vi "Autonomous Independent.vi"   [LabVIEW 2023]
doc: "This VI is called when autonomous begins, and will automatically be terminated when autonomous ends. You can carry out timed or sensor driven robot movement independently without needing to return to the caller."
uses:
  Shoulder/ShoulderGetSetpointEnum.ctl
  Auton Main/State Machine/Auot FIFO.ctl
  Auton Main/Auton Main Array.ctl
  Auton Main/State Machine/FIFO Array.ctl
  <vilib>/Rock Robotics/WPI/ThirdParty/JAS_Junk/TrajLib/Trajectory_Library.lvlib
  Auton Main/State Machine/Auot States.ctl
  Trajectory/TrajectoryGlobals.vi
  <vilib>/Rock Robotics/Network Tables/NT Read String.vi
  <vilib>/Rock Robotics/Network Tables/NT Write Number.vi
panel:
  # "Be sure to right-click and choose Data Operations>>Make Current Value default if you want to save the array values with the VI"
types:
  T1 = typedef "ShoulderGetSetpointEnum.ctl" = enum16{"Select", "ShoulderRest", "ShoulderSpeaker", "ShoulderAmp"}
  T2 = typedef "Auot States.ctl" = enum16{"Unknown", "Initilize", "Intake", "Move Arm", "Drive Straight", "Drive Trajorctory", "Drive Turn", "Send Bool CMD", "Set Target", "Shoot", "Wait", "Exit"}
  T3 = typedef "FIFO Array.ctl" = T4[]
  T4 = typedef "Auot FIFO.ctl" = cluster{"Auto States":T2, "Dist":dbl, "Radians":dbl, "MaxSpeed (ft/s)":dbl, "TimeOut (s)":dbl, "CMD":string, "ArmSetpoints":T1}
  T5 = typedef "Auton Main Array.ctl" = cluster{"FIFO Array":T3, "Dist (ft)":dbl, "MaxSpeed (ft/s)":dbl, "TimeOut (s)":dbl, "Timer Value":u32, "DriveStraightDistance":dbl[], "ModuleTravelPosition":dbl[], "First Time":bool, "Current Step":T4}
  T6 = typedef "Trajectory_Library.lvlib/TRAJECTORY.ctl" = cluster{"TotalTImeSecs":dbl, "States":T7[]}
  T7 = typedef "Trajectory_Library.lvlib/TRAJ_STATE.ctl" = cluster{"TimeSeconds":dbl, "Velocity":dbl, "Acceleration":dbl, "POSE":T8, "Curvature":dbl}
  T8 = typedef "Trajectory_Library.lvlib/POSE2D.ctl" = cluster{"TRANSLATION":T9, "ROTATION":T10}
  T9 = typedef "Trajectory_Library.lvlib/TRANSLATION2D.ctl" = cluster{"X":dbl, "Y":dbl}
  T10 = typedef "Trajectory_Library.lvlib/ROTATION2D.ctl" = cluster{"VALUE":dbl, "COS":dbl, "SIN":dbl}
  T11 = typedef "Trajectory_Library.lvlib/CHASSIS_SPEEDS.ctl" = cluster{"vX":dbl, "vY":dbl, "vOmega":dbl}
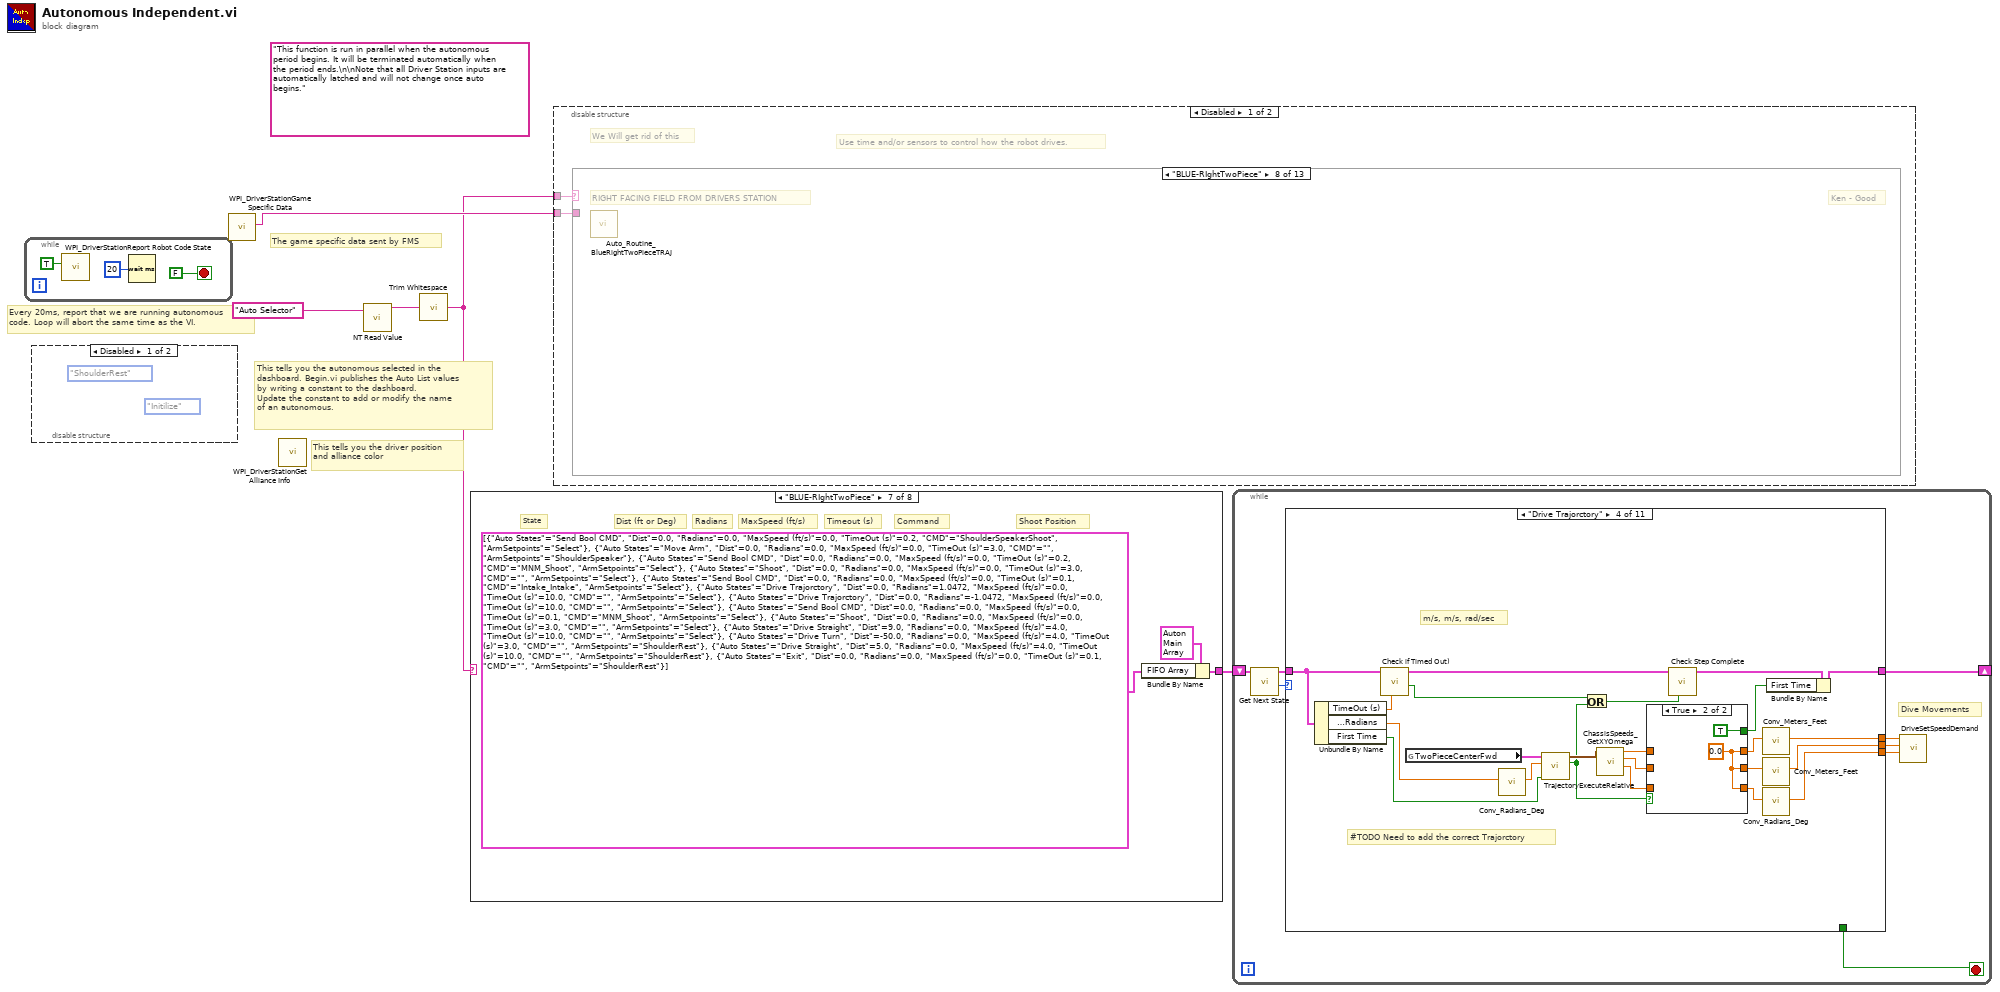
[diagram p0: block diagram]
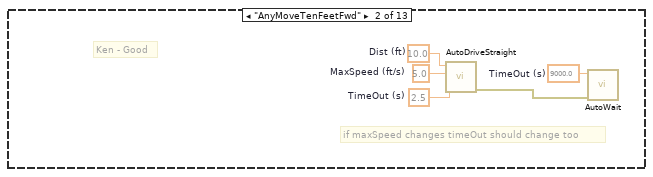
[diagram p3: hidden frame]
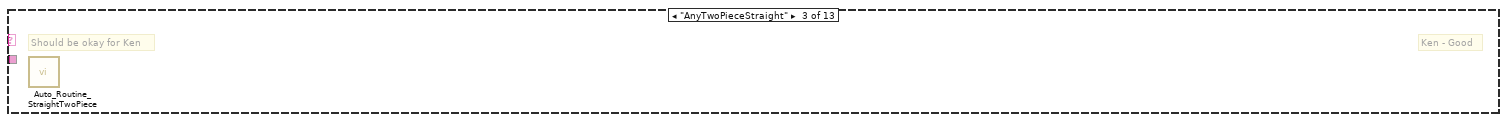
[diagram p4: hidden frame]
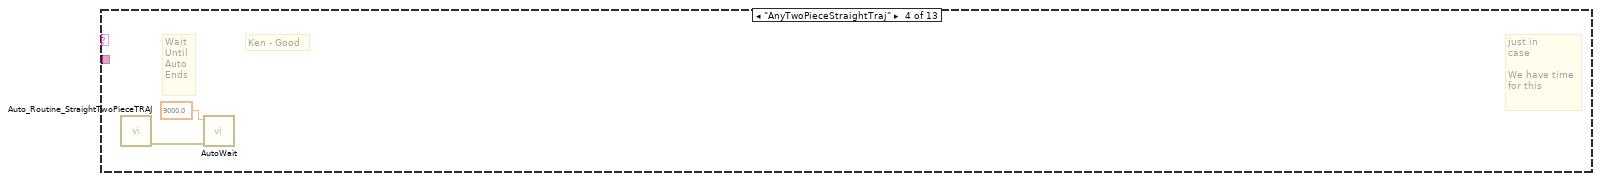
[diagram p5: hidden frame]
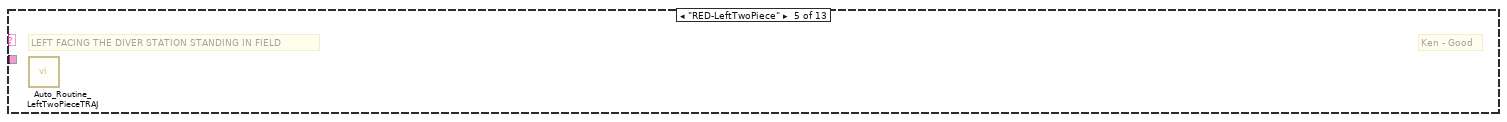
[diagram p6: hidden frame]
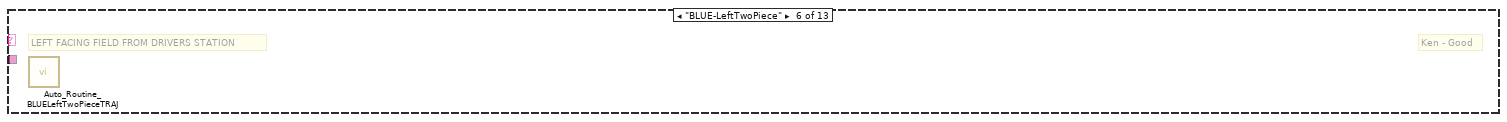
[diagram p7: hidden frame]
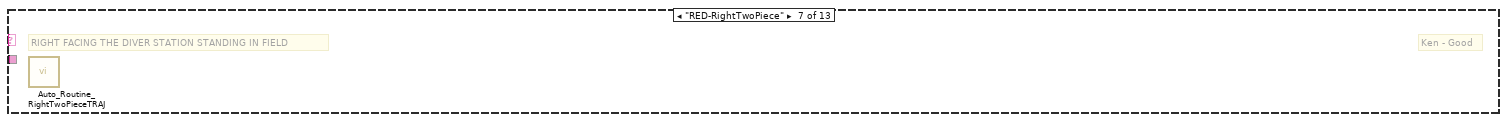
[diagram p8: hidden frame]
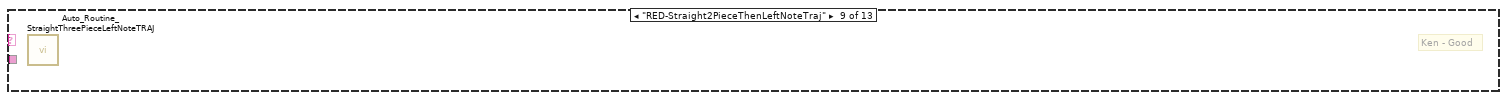
[diagram p9: hidden frame]
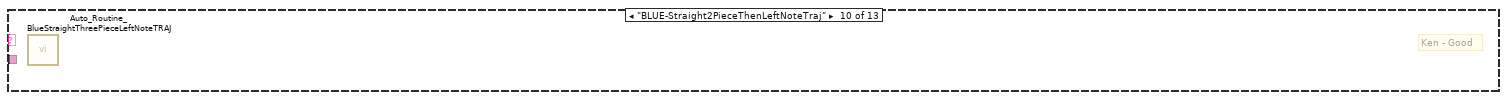
[diagram p10: hidden frame]
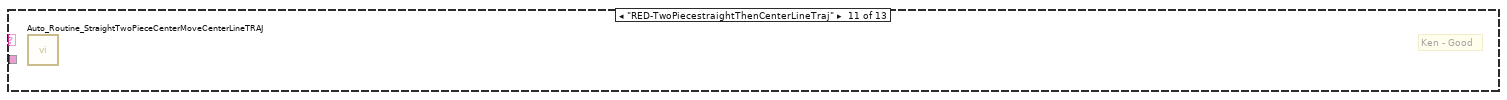
[diagram p11: hidden frame]
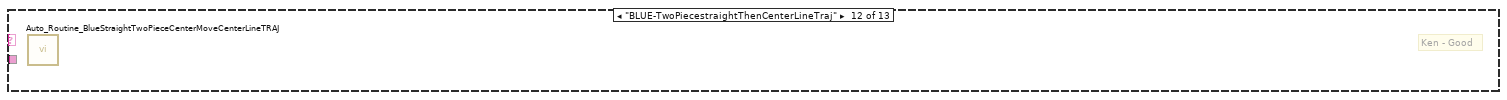
[diagram p12: hidden frame]
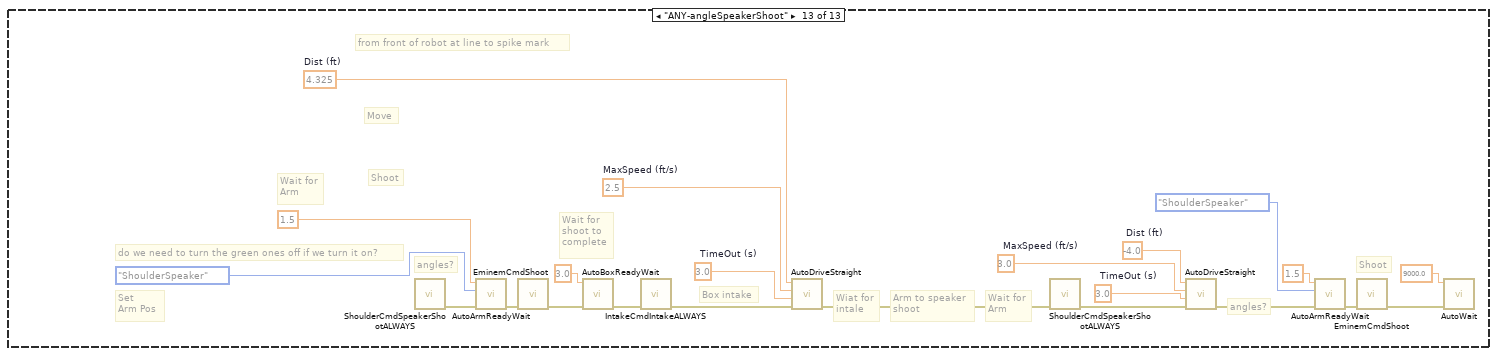
[diagram p13: hidden frame]
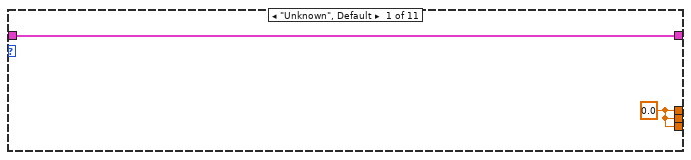
[diagram p16: hidden frame]
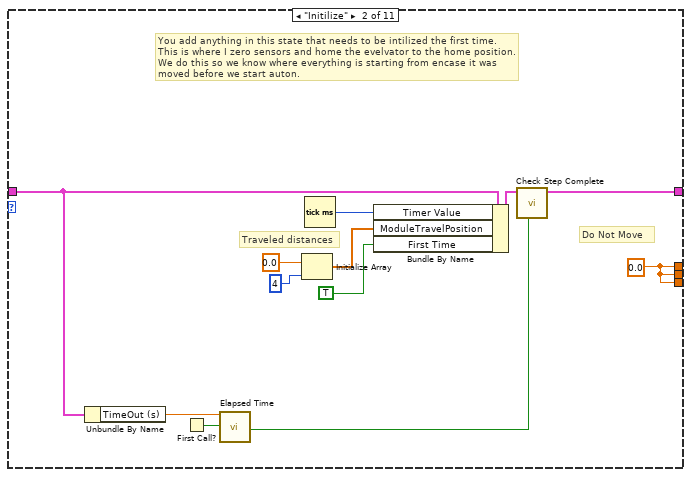
[diagram p17: hidden frame]
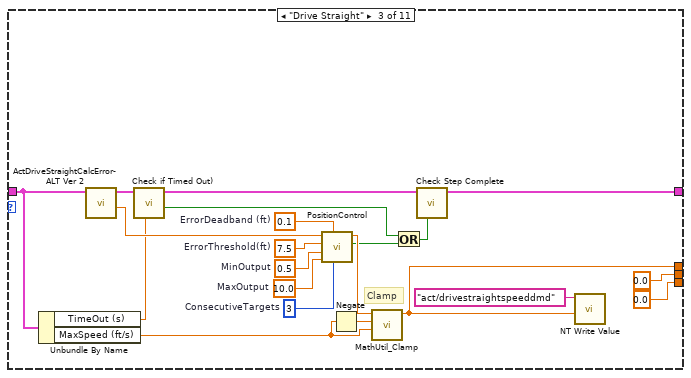
[diagram p18: hidden frame]
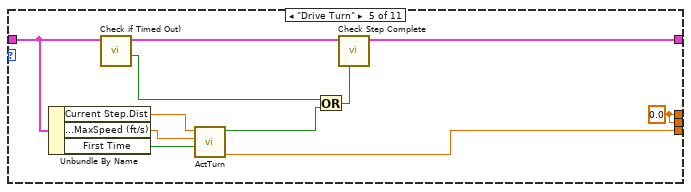
[diagram p20: hidden frame]
diagram:
  (unwired) "This function is run in parallel when the autonomous period begins. It will be terminated automatically when the period ends.\n\nNote that all Driver Station inputs are automatically latched and will not change once auto begins."
  # "The game specific data sent by FMS"
  # "This tells you the autonomous selected in the \ndashboard. Begin.vi publishes the Auto List values\nby writing a constant to the dashboard.\nUpdate the constant to add or modify the name\nof an autonomous."
  # "Every 20ms, report that we are running autonomous\ncode. Loop will abort the same time as the VI."
  # "This tells you the driver position\nand alliance color"
  n1 = while {
    stop <- FALSE stop-if-true
    n2 = call <vilib>:"WPI_DriverStationReport Robot Code State.vi"("Autonomous"=TRUE) -> ()  [unwired: 10 in, 1 out]
    n3 = Wait (ms)(milliseconds to wait=u32 20) -> ()  [unwired: 1 out]
  }
  n4 = disable-structure shown="Disabled" {
    frame Disabled {
      (unwired) ShoulderGetSetpointEnum."ShoulderRest" ("ArmSetpoints")
      (unwired) Auot_States."Initilize" ("Auto States")
    }
    frame Enabled {
    }
  }
  n5 = call <vilib>:"WPI_DriverStationGame Specific Data.vi"() -> ("Game Specific Data"=w4:string)  [unwired: 11 in]
  n6 = call <vilib>:"WPI_DriverStationGet Alliance Info.vi"() -> ()  [unwired: 12 out]
  n7 = call-poly <vilib>:"NT Read Value.vi"("name"="Auto Selector" ("Name")) -> ("value"=w3:string)  [unwired: 8 in, 2 out]
  n8 = call <vilib>:"Trim Whitespace.vi"("string"=w3) -> ("trimmed string"=w2:string)  [unwired: 1 in]
  n9 = case shown="\"BLUE-RIghtTwoPiece\"" w2 {
    tunnel: [w10 w13 w16 w19 w22 w25 w28 T5 {"FIFO Array"=[{"Auto States"=enum."Initilize", "Dist"=4.3, "Radians"=0.0, "MaxSpeed (ft/s)"=1.2, "TimeOut (s)"=10.0, "CMD"="", "ArmSetpoints"=enum."Select"}], "Dist (ft)"=0.0, "MaxSpeed (ft/s)"=0.0, "TimeOut (s)"=99.0, "Timer Value"=0, "DriveStraightDistance"=[], "ModuleTravelPosition"=[], "First Time"=FALSE, "Current Step"={"Auto States"=enum."Unknown", "Dist"=4.3, "Radians"=0.0, "MaxSpeed (ft/s)"=1.2, "TimeOut (s)"=10.0, "CMD"="", "ArmSetpoints"=enum."ShoulderRest"}} ("Main Array")] -> w1
    frame "AnyMoveTenFeetFwd" {
      # "Radians"
      # "Shoot Position"
      # "Command"
      # "Timeout (s)"
      # "MaxSpeed (ft/s)"
      # "Dist (ft)"
      # "State"
      n10 = Bundle By Name(cluster=T5 {"FIFO Array"=[{"Auto States"=enum."Initilize", "Dist"=4.3, "Radians"=0.0, "MaxSpeed (ft/s)"=1.2, "TimeOut (s)"=10.0, "CMD"="", "ArmSetpoints"=enum."ShoulderRest"}], "Dist (ft)"=0.0, "MaxSpeed (ft/s)"=0.0, "TimeOut (s)"=99.0, "Timer Value"=0, "DriveStraightDistance"=[], "ModuleTravelPosition"=[0.0, 0.0, 0.0, 0.0], "First Time"=FALSE, "Current Step"={"Auto States"=enum."Unknown", "Dist"=4.3, "Radians"=0.0, "MaxSpeed (ft/s)"=1.2, "TimeOut (s)"=10.0, "CMD"="", "ArmSetpoints"=enum."ShoulderRest"}} ("Main Array"), "FIFO Array"=T3 [{"Auto States"=enum."Initilize", "Dist"=0.0, "Radians"=0.0, "MaxSpeed (ft/s)"=0.0, "TimeOut (s)"=1.0, "CMD"="", "ArmSetpoints"=enum."Select"}, {"Auto States"=enum."Drive Straight", "Dist"=10.0, "Radians"=0.0, "MaxSpeed (ft/s)"=5.0, "TimeOut (s)"=2.5, "CMD"="", "ArmSetpoints"=enum."Select"}, {"Auto States"=enum."Exit", "Dist"=0.0, "Radians"=0.0, "MaxSpeed (ft/s)"=0.0, "TimeOut (s)"=0.1, "CMD"="", "ArmSetpoints"=enum."Select"}]) -> (w10:T5)
    }
    frame "AnyTwoPieceStraight" {
      # "Radians"
      # "Shoot Position"
      # "Command"
      # "Timeout (s)"
      # "MaxSpeed (ft/s)"
      # "Dist (ft)"
      # "State"
      n11 = Bundle By Name(cluster=T5 {"FIFO Array"=[{"Auto States"=enum."Initilize", "Dist"=0.0, "Radians"=0.0, "MaxSpeed (ft/s)"=0.0, "TimeOut (s)"=0.0, "CMD"="", "ArmSetpoints"=enum."ShoulderRest"}], "Dist (ft)"=0.0, "MaxSpeed (ft/s)"=0.0, "TimeOut (s)"=99.0, "Timer Value"=0, "DriveStraightDistance"=[], "ModuleTravelPosition"=[0.0, 0.0, 0.0, 0.0], "First Time"=FALSE, "Current Step"={"Auto States"=enum."Unknown", "Dist"=4.3, "Radians"=0.0, "MaxSpeed (ft/s)"=1.2, "TimeOut (s)"=10.0, "CMD"="", "ArmSetpoints"=enum."ShoulderRest"}} ("Main Array"), "FIFO Array"=T3 [{"Auto States"=enum."Initilize", "Dist"=0.0, "Radians"=0.0, "MaxSpeed (ft/s)"=0.0, "TimeOut (s)"=1.0, "CMD"="", "ArmSetpoints"=enum."Select"}, {"Auto States"=enum."Send Bool CMD", "Dist"=0.0, "Radians"=0.0, "MaxSpeed (ft/s)"=0.0, "TimeOut (s)"=0.2, "CMD"="ShoulderSpeakerShoot", "ArmSetpoints"=enum."Select"}, {"Auto States"=enum."Move Arm", "Dist"=0.0, "Radians"=0.0, "MaxSpeed (ft/s)"=0.0, "TimeOut (s)"=0.5, "CMD"="", "ArmSetpoints"=enum."ShoulderSpeaker"}, {"Auto States"=enum."Send Bool CMD", "Dist"=0.0, "Radians"=0.0, "MaxSpeed (ft/s)"=0.0, "TimeOut (s)"=0.2, "CMD"="MNM_Shoot", "ArmSetpoints"=enum."Select"}, {"Auto States"=enum."Shoot", "Dist"=0.0, "Radians"=0.0, "MaxSpeed (ft/s)"=0.0, "TimeOut (s)"=3.0, "CMD"="", "ArmSetpoints"=enum."Select"}, {"Auto States"=enum."Send Bool CMD", "Dist"=0.0, "Radians"=0.0, "MaxSpeed (ft/s)"=0.0, "TimeOut (s)"=0.2, "CMD"="Intake_Intake", "ArmSetpoints"=enum."Select"}, {"Auto States"=enum."Drive Straight", "Dist"=4.3, "Radians"=0.0, "MaxSpeed (ft/s)"=1.2, "TimeOut (s)"=10.0, "CMD"="", "ArmSetpoints"=enum."Select"}, {"Auto States"=enum."Drive Straight", "Dist"=-4.0, "Radians"=0.0, "MaxSpeed (ft/s)"=3.0, "TimeOut (s)"=3.0, "CMD"="", "ArmSetpoints"=enum."Select"}, {"Auto States"=enum."Send Bool CMD", "Dist"=0.0, "Radians"=0.0, "MaxSpeed (ft/s)"=0.0, "TimeOut (s)"=0.2, "CMD"="MNM_Shoot", "ArmSetpoints"=enum."Select"}, {"Auto States"=enum."Shoot", "Dist"=0.0, "Radians"=0.0, "MaxSpeed (ft/s)"=0.0, "TimeOut (s)"=3.0, "CMD"="", "ArmSetpoints"=enum."Select"}, {"Auto States"=enum."Drive Straight", "Dist"=4.0, "Radians"=0.0, "MaxSpeed (ft/s)"=3.0, "TimeOut (s)"=8.0, "CMD"="", "ArmSetpoints"=enum."Select"}, {"Auto States"=enum."Exit", "Dist"=0.0, "Radians"=0.0, "MaxSpeed (ft/s)"=0.0, "TimeOut (s)"=0.1, "CMD"="", "ArmSetpoints"=enum."Select"}]) -> (w13:T5)
    }
    frame "AnyTwoPieceStraightTraj" {
      # "Radians"
      # "Shoot Position"
      # "Command"
      # "Timeout (s)"
      # "MaxSpeed (ft/s)"
      # "Dist (ft)"
      # "State"
      n12 = Bundle By Name(cluster=T5 {"FIFO Array"=[{"Auto States"=enum."Initilize", "Dist"=0.0, "Radians"=0.0, "MaxSpeed (ft/s)"=0.0, "TimeOut (s)"=0.0, "CMD"="", "ArmSetpoints"=enum."ShoulderRest"}], "Dist (ft)"=0.0, "MaxSpeed (ft/s)"=0.0, "TimeOut (s)"=99.0, "Timer Value"=0, "DriveStraightDistance"=[], "ModuleTravelPosition"=[0.0, 0.0, 0.0, 0.0], "First Time"=FALSE, "Current Step"={"Auto States"=enum."Unknown", "Dist"=4.3, "Radians"=0.0, "MaxSpeed (ft/s)"=1.2, "TimeOut (s)"=10.0, "CMD"="", "ArmSetpoints"=enum."ShoulderRest"}} ("Main Array"), "FIFO Array"=T3 [{"Auto States"=enum."Initilize", "Dist"=0.0, "Radians"=0.0, "MaxSpeed (ft/s)"=0.0, "TimeOut (s)"=0.1, "CMD"="", "ArmSetpoints"=enum."Select"}, {"Auto States"=enum."Send Bool CMD", "Dist"=0.0, "Radians"=0.0, "MaxSpeed (ft/s)"=0.0, "TimeOut (s)"=0.2, "CMD"="ShoulderSpeakerShoot", "ArmSetpoints"=enum."Select"}, {"Auto States"=enum."Send Bool CMD", "Dist"=0.0, "Radians"=0.0, "MaxSpeed (ft/s)"=0.0, "TimeOut (s)"=0.2, "CMD"="MNM_ShootRev", "ArmSetpoints"=enum."Select"}, {"Auto States"=enum."Move Arm", "Dist"=0.0, "Radians"=0.0, "MaxSpeed (ft/s)"=0.0, "TimeOut (s)"=1.5, "CMD"="", "ArmSetpoints"=enum."ShoulderSpeaker"}, {"Auto States"=enum."Send Bool CMD", "Dist"=0.0, "Radians"=0.0, "MaxSpeed (ft/s)"=0.0, "TimeOut (s)"=0.2, "CMD"="MNM_Shoot", "ArmSetpoints"=enum."Select"}, {"Auto States"=enum."Shoot", "Dist"=0.0, "Radians"=0.0, "MaxSpeed (ft/s)"=0.0, "TimeOut (s)"=3.0, "CMD"="", "ArmSetpoints"=enum."Select"}, {"Auto States"=enum."Send Bool CMD", "Dist"=0.0, "Radians"=0.0, "MaxSpeed (ft/s)"=0.0, "TimeOut (s)"=0.2, "CMD"="Intake_Intake", "ArmSetpoints"=enum."Select"}, {"Auto States"=enum."Drive Trajorctory", "Dist"=0.0, "Radians"=0.0, "MaxSpeed (ft/s)"=0.0, "TimeOut (s)"=10.0, "CMD"="", "ArmSetpoints"=enum."Select"}, {"Auto States"=enum."Wait", "Dist"=0.0, "Radians"=0.0, "MaxSpeed (ft/s)"=0.0, "TimeOut (s)"=0.1, "CMD"="", "ArmSetpoints"=enum."Select"}, {"Auto States"=enum."Drive Trajorctory", "Dist"=0.0, "Radians"=0.0, "MaxSpeed (ft/s)"=0.0, "TimeOut (s)"=2.8, "CMD"="", "ArmSetpoints"=enum."Select"}, {"Auto States"=enum."Send Bool CMD", "Dist"=0.0, "Radians"=0.0, "MaxSpeed (ft/s)"=0.0, "TimeOut (s)"=0.2, "CMD"="MNM_ShootRev", "ArmSetpoints"=enum."Select"}, {"Auto States"=enum."Send Bool CMD", "Dist"=0.0, "Radians"=0.0, "MaxSpeed (ft/s)"=0.0, "TimeOut (s)"=0.2, "CMD"="MNM_Shoot", "ArmSetpoints"=enum."Select"}, {"Auto States"=enum."Shoot", "Dist"=0.0, "Radians"=0.0, "MaxSpeed (ft/s)"=0.0, "TimeOut (s)"=3.0, "CMD"="", "ArmSetpoints"=enum."Select"}, {"Auto States"=enum."Exit", "Dist"=0.0, "Radians"=0.0, "MaxSpeed (ft/s)"=0.0, "TimeOut (s)"=0.1, "CMD"="", "ArmSetpoints"=enum."Select"}]) -> (w16:T5)
    }
    frame "RED-LeftTwoPiece" {
      # "Radians"
      # "Shoot Position"
      # "Command"
      # "Timeout (s)"
      # "MaxSpeed (ft/s)"
      # "Dist (ft)"
      # "State"
      n13 = Bundle By Name(cluster=T5 {"FIFO Array"=[{"Auto States"=enum."Unknown", "Dist"=0.0, "Radians"=0.0, "MaxSpeed (ft/s)"=0.0, "TimeOut (s)"=0.1, "CMD"="", "ArmSetpoints"=enum."Select"}], "Dist (ft)"=0.0, "MaxSpeed (ft/s)"=0.0, "TimeOut (s)"=99.0, "Timer Value"=0, "DriveStraightDistance"=[], "ModuleTravelPosition"=[0.0, 0.0, 0.0, 0.0], "First Time"=FALSE, "Current Step"={"Auto States"=enum."Unknown", "Dist"=4.3, "Radians"=0.0, "MaxSpeed (ft/s)"=1.2, "TimeOut (s)"=10.0, "CMD"="", "ArmSetpoints"=enum."ShoulderRest"}} ("Main Array"), "FIFO Array"=T3 [{"Auto States"=enum."Send Bool CMD", "Dist"=0.0, "Radians"=0.0, "MaxSpeed (ft/s)"=0.0, "TimeOut (s)"=0.2, "CMD"="ShoulderSpeakerShoot", "ArmSetpoints"=enum."Select"}, {"Auto States"=enum."Move Arm", "Dist"=0.0, "Radians"=0.0, "MaxSpeed (ft/s)"=0.0, "TimeOut (s)"=3.0, "CMD"="", "ArmSetpoints"=enum."ShoulderSpeaker"}, {"Auto States"=enum."Send Bool CMD", "Dist"=0.0, "Radians"=0.0, "MaxSpeed (ft/s)"=0.0, "TimeOut (s)"=0.2, "CMD"="MNM_Shoot", "ArmSetpoints"=enum."Select"}, {"Auto States"=enum."Shoot", "Dist"=0.0, "Radians"=0.0, "MaxSpeed (ft/s)"=0.0, "TimeOut (s)"=3.0, "CMD"="", "ArmSetpoints"=enum."Select"}, {"Auto States"=enum."Send Bool CMD", "Dist"=0.0, "Radians"=0.0, "MaxSpeed (ft/s)"=0.0, "TimeOut (s)"=0.1, "CMD"="Intake_Intake", "ArmSetpoints"=enum."Select"}, {"Auto States"=enum."Drive Trajorctory", "Dist"=0.0, "Radians"=1.0472, "MaxSpeed (ft/s)"=0.0, "TimeOut (s)"=10.0, "CMD"="", "ArmSetpoints"=enum."Select"}, {"Auto States"=enum."Drive Trajorctory", "Dist"=0.0, "Radians"=-1.0472, "MaxSpeed (ft/s)"=0.0, "TimeOut (s)"=10.0, "CMD"="", "ArmSetpoints"=enum."Select"}, {"Auto States"=enum."Send Bool CMD", "Dist"=0.0, "Radians"=0.0, "MaxSpeed (ft/s)"=0.0, "TimeOut (s)"=0.1, "CMD"="MNM_Shoot", "ArmSetpoints"=enum."Select"}, {"Auto States"=enum."Shoot", "Dist"=0.0, "Radians"=0.0, "MaxSpeed (ft/s)"=0.0, "TimeOut (s)"=3.0, "CMD"="", "ArmSetpoints"=enum."Select"}, {"Auto States"=enum."Exit", "Dist"=0.0, "Radians"=0.0, "MaxSpeed (ft/s)"=0.0, "TimeOut (s)"=0.1, "CMD"="", "ArmSetpoints"=enum."Select"}]) -> (w19:T5)
    }
    frame "BLUE-LeftTwoPiece" {
      # "Radians"
      # "Shoot Position"
      # "Command"
      # "Timeout (s)"
      # "MaxSpeed (ft/s)"
      # "Dist (ft)"
      # "State"
      n14 = Bundle By Name(cluster=T5 {"FIFO Array"=[{"Auto States"=enum."Unknown", "Dist"=0.0, "Radians"=0.0, "MaxSpeed (ft/s)"=0.0, "TimeOut (s)"=0.1, "CMD"="", "ArmSetpoints"=enum."Select"}], "Dist (ft)"=0.0, "MaxSpeed (ft/s)"=0.0, "TimeOut (s)"=99.0, "Timer Value"=0, "DriveStraightDistance"=[], "ModuleTravelPosition"=[0.0, 0.0, 0.0, 0.0], "First Time"=FALSE, "Current Step"={"Auto States"=enum."Unknown", "Dist"=4.3, "Radians"=0.0, "MaxSpeed (ft/s)"=1.2, "TimeOut (s)"=10.0, "CMD"="", "ArmSetpoints"=enum."ShoulderRest"}} ("Main Array"), "FIFO Array"=T3 [{"Auto States"=enum."Send Bool CMD", "Dist"=0.0, "Radians"=0.0, "MaxSpeed (ft/s)"=0.0, "TimeOut (s)"=0.2, "CMD"="ShoulderSpeakerShoot", "ArmSetpoints"=enum."Select"}, {"Auto States"=enum."Move Arm", "Dist"=0.0, "Radians"=0.0, "MaxSpeed (ft/s)"=0.0, "TimeOut (s)"=3.0, "CMD"="", "ArmSetpoints"=enum."ShoulderSpeaker"}, {"Auto States"=enum."Send Bool CMD", "Dist"=0.0, "Radians"=0.0, "MaxSpeed (ft/s)"=0.0, "TimeOut (s)"=0.2, "CMD"="MNM_Shoot", "ArmSetpoints"=enum."Select"}, {"Auto States"=enum."Shoot", "Dist"=0.0, "Radians"=0.0, "MaxSpeed (ft/s)"=0.0, "TimeOut (s)"=3.0, "CMD"="", "ArmSetpoints"=enum."Select"}, {"Auto States"=enum."Send Bool CMD", "Dist"=0.0, "Radians"=0.0, "MaxSpeed (ft/s)"=0.0, "TimeOut (s)"=0.1, "CMD"="Intake_Intake", "ArmSetpoints"=enum."Select"}, {"Auto States"=enum."Drive Trajorctory", "Dist"=0.0, "Radians"=-1.0472, "MaxSpeed (ft/s)"=0.0, "TimeOut (s)"=10.0, "CMD"="", "ArmSetpoints"=enum."Select"}, {"Auto States"=enum."Drive Trajorctory", "Dist"=0.0, "Radians"=1.0472, "MaxSpeed (ft/s)"=0.0, "TimeOut (s)"=10.0, "CMD"="", "ArmSetpoints"=enum."Select"}, {"Auto States"=enum."Send Bool CMD", "Dist"=0.0, "Radians"=0.0, "MaxSpeed (ft/s)"=0.0, "TimeOut (s)"=0.1, "CMD"="MNM_Shoot", "ArmSetpoints"=enum."Select"}, {"Auto States"=enum."Shoot", "Dist"=0.0, "Radians"=0.0, "MaxSpeed (ft/s)"=0.0, "TimeOut (s)"=3.0, "CMD"="", "ArmSetpoints"=enum."Select"}, {"Auto States"=enum."Exit", "Dist"=0.0, "Radians"=0.0, "MaxSpeed (ft/s)"=0.0, "TimeOut (s)"=0.1, "CMD"="", "ArmSetpoints"=enum."Select"}]) -> (w22:T5)
    }
    frame "RED-RightTwoPiece" {
      # "Radians"
      # "Shoot Position"
      # "Command"
      # "Timeout (s)"
      # "MaxSpeed (ft/s)"
      # "Dist (ft or Deg)"
      # "State"
      n15 = Bundle By Name(cluster=T5 {"FIFO Array"=[{"Auto States"=enum."Unknown", "Dist"=0.0, "Radians"=0.0, "MaxSpeed (ft/s)"=0.0, "TimeOut (s)"=0.1, "CMD"="", "ArmSetpoints"=enum."Select"}], "Dist (ft)"=0.0, "MaxSpeed (ft/s)"=0.0, "TimeOut (s)"=99.0, "Timer Value"=0, "DriveStraightDistance"=[], "ModuleTravelPosition"=[0.0, 0.0, 0.0, 0.0], "First Time"=FALSE, "Current Step"={"Auto States"=enum."Unknown", "Dist"=4.3, "Radians"=0.0, "MaxSpeed (ft/s)"=1.2, "TimeOut (s)"=10.0, "CMD"="", "ArmSetpoints"=enum."ShoulderRest"}} ("Main Array"), "FIFO Array"=T3 [{"Auto States"=enum."Send Bool CMD", "Dist"=0.0, "Radians"=0.0, "MaxSpeed (ft/s)"=0.0, "TimeOut (s)"=0.2, "CMD"="ShoulderSpeakerShoot", "ArmSetpoints"=enum."Select"}, {"Auto States"=enum."Move Arm", "Dist"=0.0, "Radians"=0.0, "MaxSpeed (ft/s)"=0.0, "TimeOut (s)"=3.0, "CMD"="", "ArmSetpoints"=enum."ShoulderSpeaker"}, {"Auto States"=enum."Send Bool CMD", "Dist"=0.0, "Radians"=0.0, "MaxSpeed (ft/s)"=0.0, "TimeOut (s)"=0.2, "CMD"="MNM_Shoot", "ArmSetpoints"=enum."Select"}, {"Auto States"=enum."Shoot", "Dist"=0.0, "Radians"=0.0, "MaxSpeed (ft/s)"=0.0, "TimeOut (s)"=3.0, "CMD"="", "ArmSetpoints"=enum."Select"}, {"Auto States"=enum."Send Bool CMD", "Dist"=0.0, "Radians"=0.0, "MaxSpeed (ft/s)"=0.0, "TimeOut (s)"=0.1, "CMD"="Intake_Intake", "ArmSetpoints"=enum."Select"}, {"Auto States"=enum."Drive Trajorctory", "Dist"=0.0, "Radians"=-1.0472, "MaxSpeed (ft/s)"=0.0, "TimeOut (s)"=10.0, "CMD"="", "ArmSetpoints"=enum."Select"}, {"Auto States"=enum."Drive Trajorctory", "Dist"=0.0, "Radians"=1.0472, "MaxSpeed (ft/s)"=0.0, "TimeOut (s)"=10.0, "CMD"="", "ArmSetpoints"=enum."Select"}, {"Auto States"=enum."Send Bool CMD", "Dist"=0.0, "Radians"=0.0, "MaxSpeed (ft/s)"=0.0, "TimeOut (s)"=0.1, "CMD"="MNM_Shoot", "ArmSetpoints"=enum."Select"}, {"Auto States"=enum."Shoot", "Dist"=0.0, "Radians"=0.0, "MaxSpeed (ft/s)"=0.0, "TimeOut (s)"=3.0, "CMD"="", "ArmSetpoints"=enum."Select"}, {"Auto States"=enum."Drive Straight", "Dist"=9.0, "Radians"=0.0, "MaxSpeed (ft/s)"=4.0, "TimeOut (s)"=10.0, "CMD"="", "ArmSetpoints"=enum."Select"}, {"Auto States"=enum."Drive Turn", "Dist"=-50.0, "Radians"=0.0, "MaxSpeed (ft/s)"=4.0, "TimeOut (s)"=3.0, "CMD"="", "ArmSetpoints"=enum."ShoulderRest"}, {"Auto States"=enum."Drive Straight", "Dist"=5.0, "Radians"=0.0, "MaxSpeed (ft/s)"=4.0, "TimeOut (s)"=10.0, "CMD"="", "ArmSetpoints"=enum."ShoulderRest"}, {"Auto States"=enum."Exit", "Dist"=0.0, "Radians"=0.0, "MaxSpeed (ft/s)"=0.0, "TimeOut (s)"=0.1, "CMD"="", "ArmSetpoints"=enum."ShoulderRest"}]) -> (w25:T5)
    }
    frame "BLUE-RIghtTwoPiece" {
      # "Radians"
      # "Shoot Position"
      # "Command"
      # "Timeout (s)"
      # "MaxSpeed (ft/s)"
      # "Dist (ft or Deg)"
      # "State"
      n16 = Bundle By Name(cluster=T5 {"FIFO Array"=[{"Auto States"=enum."Unknown", "Dist"=0.0, "Radians"=0.0, "MaxSpeed (ft/s)"=0.0, "TimeOut (s)"=0.1, "CMD"="", "ArmSetpoints"=enum."Select"}], "Dist (ft)"=0.0, "MaxSpeed (ft/s)"=0.0, "TimeOut (s)"=99.0, "Timer Value"=0, "DriveStraightDistance"=[], "ModuleTravelPosition"=[0.0, 0.0, 0.0, 0.0], "First Time"=FALSE, "Current Step"={"Auto States"=enum."Unknown", "Dist"=4.3, "Radians"=0.0, "MaxSpeed (ft/s)"=1.2, "TimeOut (s)"=10.0, "CMD"="", "ArmSetpoints"=enum."ShoulderRest"}} ("Main Array"), "FIFO Array"=T3 [{"Auto States"=enum."Send Bool CMD", "Dist"=0.0, "Radians"=0.0, "MaxSpeed (ft/s)"=0.0, "TimeOut (s)"=0.2, "CMD"="ShoulderSpeakerShoot", "ArmSetpoints"=enum."Select"}, {"Auto States"=enum."Move Arm", "Dist"=0.0, "Radians"=0.0, "MaxSpeed (ft/s)"=0.0, "TimeOut (s)"=3.0, "CMD"="", "ArmSetpoints"=enum."ShoulderSpeaker"}, {"Auto States"=enum."Send Bool CMD", "Dist"=0.0, "Radians"=0.0, "MaxSpeed (ft/s)"=0.0, "TimeOut (s)"=0.2, "CMD"="MNM_Shoot", "ArmSetpoints"=enum."Select"}, {"Auto States"=enum."Shoot", "Dist"=0.0, "Radians"=0.0, "MaxSpeed (ft/s)"=0.0, "TimeOut (s)"=3.0, "CMD"="", "ArmSetpoints"=enum."Select"}, {"Auto States"=enum."Send Bool CMD", "Dist"=0.0, "Radians"=0.0, "MaxSpeed (ft/s)"=0.0, "TimeOut (s)"=0.1, "CMD"="Intake_Intake", "ArmSetpoints"=enum."Select"}, {"Auto States"=enum."Drive Trajorctory", "Dist"=0.0, "Radians"=1.0472, "MaxSpeed (ft/s)"=0.0, "TimeOut (s)"=10.0, "CMD"="", "ArmSetpoints"=enum."Select"}, {"Auto States"=enum."Drive Trajorctory", "Dist"=0.0, "Radians"=-1.0472, "MaxSpeed (ft/s)"=0.0, "TimeOut (s)"=10.0, "CMD"="", "ArmSetpoints"=enum."Select"}, {"Auto States"=enum."Send Bool CMD", "Dist"=0.0, "Radians"=0.0, "MaxSpeed (ft/s)"=0.0, "TimeOut (s)"=0.1, "CMD"="MNM_Shoot", "ArmSetpoints"=enum."Select"}, {"Auto States"=enum."Shoot", "Dist"=0.0, "Radians"=0.0, "MaxSpeed (ft/s)"=0.0, "TimeOut (s)"=3.0, "CMD"="", "ArmSetpoints"=enum."Select"}, {"Auto States"=enum."Drive Straight", "Dist"=9.0, "Radians"=0.0, "MaxSpeed (ft/s)"=4.0, "TimeOut (s)"=10.0, "CMD"="", "ArmSetpoints"=enum."Select"}, {"Auto States"=enum."Drive Turn", "Dist"=-50.0, "Radians"=0.0, "MaxSpeed (ft/s)"=4.0, "TimeOut (s)"=3.0, "CMD"="", "ArmSetpoints"=enum."ShoulderRest"}, {"Auto States"=enum."Drive Straight", "Dist"=5.0, "Radians"=0.0, "MaxSpeed (ft/s)"=4.0, "TimeOut (s)"=10.0, "CMD"="", "ArmSetpoints"=enum."ShoulderRest"}, {"Auto States"=enum."Exit", "Dist"=0.0, "Radians"=0.0, "MaxSpeed (ft/s)"=0.0, "TimeOut (s)"=0.1, "CMD"="", "ArmSetpoints"=enum."ShoulderRest"}]) -> (w28:T5)
    }
    frame Default {
    }
  }
  n17 = disable-structure shown="Disabled" {
    disable-tunnel: w4 -> [w32 _]
    disable-tunnel: w2 -> [w31 _]
    frame Disabled {
      # "We Will get rid of this"
      # "Use time and/or sensors to control how the robot drives."
      n18 = case shown="\"BLUE-RIghtTwoPiece\"" w31 {
        tunnel: w32 -> [_ _ _ _ _ _ _ _ _ _ _ _ _]
        frame Default {
          # "You can put your main auto here, or you can right-click on the case and make any\nother frame be the default case."
          # "This is the frame that will execute if no selection is made, or if it is not recognized"
        }
        frame "AnyMoveTenFeetFwd" {
          w33 = 9000.0  # TimeOut (s)
          w35 = 2.5  # TimeOut (s)
          w36 = 5.0  # MaxSpeed (ft/s)
          w37 = 10.0  # Dist (ft)
          # "Ken - Good"
          # "if maxSpeed changes timeOut should change too"
          n19 = call "AutoDriveStraight.vi"("TimeOut (s)"=w35, "MaxSpeed (ft/s)"=w36, "Dist (ft)"=w37) -> ("error out"=w34:errorcluster)  [unwired: 8 in]
          n20 = call "AutoWait.vi"("error in (no error)"=w34, "TimeOut (s)"=w33) -> ()  [unwired: 9 in, 1 out]
        }
        frame "AnyTwoPieceStraight" {
          # "Ken - Good"
          # "Should be okay for Ken"
          n21 = call "Auto_Routine_StraightTwoPiece.vi"() -> ()  [unwired: 11 in, 1 out]
        }
        frame "AnyTwoPieceStraightTraj" {
          # "Ken - Good"
          # "just in\ncase\n\nWe have time\nfor this"
          # "Wait\nUntil\nAuto \nEnds"
          n22 = call "Auto_Routine_StraightTwoPieceTRAJ.vi"() -> ("error out"=w38:errorcluster)  [unwired: 11 in]
          n23 = call "AutoWait.vi"("error in (no error)"=w38, "TimeOut (s)"=9000.0) -> ()  [unwired: 9 in, 1 out]
        }
        frame "RED-LeftTwoPiece" {
          # "Ken - Good"
          # "LEFT FACING THE DIVER STATION STANDING IN FIELD"
          n24 = call "Auto_Routine_LeftTwoPieceTRAJ.vi"() -> ()  [unwired: 12 in]
        }
        frame "BLUE-LeftTwoPiece" {
          # "Ken - Good"
          # "LEFT FACING FIELD FROM DRIVERS STATION"
          n25 = call "Auto_Routine_BLUELeftTwoPieceTRAJ.vi"() -> ()  [unwired: 12 in]
        }
        frame "RED-RightTwoPiece" {
          # "Ken - Good"
          # "RIGHT FACING THE DIVER STATION STANDING IN FIELD"
          n26 = call "Auto_Routine_RightTwoPieceTRAJ.vi"() -> ()  [unwired: 12 in]
        }
        frame "BLUE-RIghtTwoPiece" {
          # "Ken - Good"
          # "RIGHT FACING FIELD FROM DRIVERS STATION"
          n27 = call "Auto_Routine_BlueRightTwoPieceTRAJ.vi"() -> ()  [unwired: 12 in]
        }
        frame "RED-Straight2PieceThenLeftNoteTraj" {
          # "Ken - Good"
          n28 = call "Auto_Routine_StraightThreePieceLeftNoteTRAJ.vi"() -> ()  [unwired: 11 in, 1 out]
        }
        frame "BLUE-Straight2PieceThenLeftNoteTraj" {
          # "Ken - Good"
          n29 = call "Auto_Routine_BlueStraightThreePieceLeftNoteTRAJ.vi"() -> ()  [unwired: 11 in, 1 out]
        }
        frame "RED-TwoPiecestraightThenCenterLineTraj" {
          # "Ken - Good"
          n30 = call "Auto_Routine_StraightTwoPieceCenterMoveCenterLineTRAJ.vi"() -> ()  [unwired: 11 in, 1 out]
        }
        frame "BLUE-TwoPiecestraightThenCenterLineTraj" {
          # "Ken - Good"
          n31 = call "Auto_Routine_BlueStraightTwoPieceCenterMoveCenterLineTRAJ.vi"() -> ()  [unwired: 11 in, 1 out]
        }
        frame "ANY-angleSpeakerShoot" {
          w47 = 3.0  # TimeOut (s)
          w48 = 3.0  # MaxSpeed (ft/s)
          w49 = -4.0  # Dist (ft)
          w59 = 3.0  # TimeOut (s)
          w60 = 2.5  # MaxSpeed (ft/s)
          w61 = 4.325  # Dist (ft)
          # "Shoot"
          # "Wait for\nArm"
          # "Arm to speaker\nshoot"
          # "Wiat for\nintale"
          # "Box intake"
          # "Move"
          # "Wait for\nshoot to\ncomplete"
          # "Shoot"
          # "Wait for\nArm"
          # "Set\nArm Pos"
          # "do we need to turn the green ones off if we turn it on?"
          # "angles?"
          # "angles?"
          # "from front of robot at line to spike mark"
          n32 = call "ShoulderCmdSpeakerShootALWAYS.vi"() -> ("error out"=w56:errorcluster)  [unwired: 11 in]
          n33 = call "AutoArmReadyWait.vi"("error in (no error)"=w56, "ArmSetpoints"=ShoulderGetSetpointEnum."ShoulderSpeaker", "TimeOut (s)"=1.5) -> ("error out"=w55:errorcluster)  [unwired: 8 in]
          n34 = call "EminemCmdShoot.vi"("error in (no error)"=w55) -> ("error out"=w53:errorcluster)  [unwired: 10 in]
          n35 = call "AutoBoxReadyWait.vi"("error in (no error)"=w53, "TimeOut (s)"=3.0) -> ("error out"=w40:errorcluster)  [unwired: 9 in]
          n36 = call "IntakeCmdIntakeALWAYS.vi"("error in (no error)"=w40) -> ("error out"=w41:errorcluster)  [unwired: 10 in]
          n37 = call "AutoDriveStraight.vi"("error in (no error)"=w41, "TimeOut (s)"=w59, "MaxSpeed (ft/s)"=w60, "Dist (ft)"=w61) -> ("error out"=w45:errorcluster)  [unwired: 7 in]
          n38 = call "ShoulderCmdSpeakerShootALWAYS.vi"("error in (no error)"=w45) -> ("error out"=w44:errorcluster)  [unwired: 10 in]
          n39 = call "AutoDriveStraight.vi"("error in (no error)"=w44, "TimeOut (s)"=w47, "MaxSpeed (ft/s)"=w48, "Dist (ft)"=w49) -> ("error out"=w46:errorcluster)  [unwired: 7 in]
          n40 = call "AutoArmReadyWait.vi"("error in (no error)"=w46, "ArmSetpoints"=ShoulderGetSetpointEnum."ShoulderSpeaker", "TimeOut (s)"=1.5) -> ("error out"=w51:errorcluster)  [unwired: 8 in]
          n41 = call "EminemCmdShoot.vi"("error in (no error)"=w51) -> ("error out"=w58:errorcluster)  [unwired: 10 in]
          n42 = call "AutoWait.vi"("error in (no error)"=w58, "TimeOut (s)"=9000.0) -> ()  [unwired: 9 in, 1 out]
        }
      }
    }
    frame Enabled {
    }
  }
  n43 = while {
    shift-right: [w66] -> _
    shift-left: w1 -> [w69]
    stop <- w62 stop-if-true
    # "Dive Movements"
    n44 = call "Get Next State.vi"("Main Array"=w69) -> ("Next State"=w68:T2, "Main Array out"=w67:T5)  [unwired: 9 in]
    n45 = case shown="\"Drive Trajorctory\"" w68 {
      tunnel: w67 -> [w71 w76 w84 w114 w141 w144 w153 w160 w161 w168 w171]
      tunnel: [w71 w81 w95 w108 w142 w151 w156 w160 w166 w168 w171] -> w66
      tunnel: [w70 w80 w93 w119 w136 w145 w154 _ _ _ w169] -> w65
      tunnel: [w70 w80 0.0 w118 w136 w145 w154 _ _ _ w169] -> w64
      tunnel: [w70 w80 0.0 w117 w137 w145 w154 _ _ _ w169] -> w63
      tunnel: [_ _ _ _ _ _ _ _ _ _ TRUE] -> w62
      frame "Unknown", Default {
        w70 = 0.0
      }
      frame "Initilize" {
        w80 = 0.0
        # "You add anything in this state that needs to be intilized the first time. This is where I zero sensors and home the evelvator to the home position. We do this so we know where everything is starting from encase it was moved before we start auton."
        # "Traveled distances"
        # "Do Not Move"
        n46 = Unbundle By Name(w76) -> ("TimeOut (s)"=w75:dbl)
        n47 = First Call?() -> (First Call?: T/F=w74:bool)
        n48 = call "Elapsed Time"("Time Target (s)"=w75, "Reset"=w74) -> ("Time has Elapsed"=w73:bool)  [unwired: 10 in, 7 out]
        n49 = Initialize Array(0.0 ("element"), 4 ("dimension size")) -> (w77:dbl[])
        n50 = Tick Count (ms)() -> (millisecond timer value=w83:u32)
        n51 = Bundle By Name(cluster=w76, "Timer Value"=w83, "ModuleTravelPosition"=w77, "First Time"=TRUE) -> (w82:T5)
        n52 = call "Check Step Complete.vi"("Move Complete"=w73, "Main Array in"=w82) -> ("Main Array iout"=w81:T5)  [unwired: 9 in]
      }
      frame "Drive Straight" {
        w98 = 10.0  # MaxOutput
        w99 = 0.5  # MinOutput
        w102 = 3  # ConsecutiveTargets
        w103 = 0.1  # ErrorDeadband (ft)
        w104 = 7.5  # ErrorThreshold(ft)
        # "Clamp"
        n53 = Unbundle By Name(w84) -> ("TimeOut (s)"=w85:dbl, "MaxSpeed (ft/s)"=w96:dbl)
        n54 = call "ActDriveStraightCalcError-ALT Ver 2.vi"("Main Array in"=w84) -> ("Dist Error (Ft)"=w94:dbl, "Main Array out"=w89:T5)  [unwired: 9 in]
        n55 = call "Check if Timed Out).vi"("Time out"=w85, "Main Array in"=w89) -> ("Timed Out"=w86:bool, "Main Array out"=w88:T5)  [unwired: 8 in]
        n56 = call "PositionControl.vi"("ConsecutiveTargets"=w102, "ErrorDeadband"=w103, "MaxOutput"=w98, "MinOutput"=w99, "ErrorThreshold"=w104, "Error"=w94) -> ("OnTarget"=w87:bool, "OutputValue"=w101:dbl)  [unwired: 3 in, 1 out]
        n57 = Negate(x=w96) -> (-x=w100:dbl)
        n58 = call <vilib>:"MathUtil_Clamp.vi"("High Limit"=w96, "Low Limit"=w100, "Value"=w101) -> ("Result"=w93:dbl)  [unwired: 8 in]
        n59 = Or(x=w86, y=w87) -> (x .or. y?=w90:bool)
        n60 = call "Check Step Complete.vi"("Move Complete"=w90, "Main Array in"=w88) -> ("Main Array iout"=w95:T5)  [unwired: 9 in]
        n61 = call-poly <vilib>:"NT Write Value.vi"("value"=w93, "name"="act/drivestraightspeeddmd") -> ()  [unwired: 9 in, 1 out]
      }
      frame "Drive Trajorctory" {
        # "#TODO Need to add the correct Trajorctory"
        # "m/s, m/s, rad/sec"
        n62 = Unbundle By Name(w114) -> ("TimeOut (s)"=w115:dbl, "Current Step.Radians"=w105:dbl, "First Time"=w106:bool)
        n63 = call "Check if Timed Out).vi"("Time out"=w115, "Main Array in"=w114) -> ("Timed Out"=w110:bool, "Main Array out"=w113:T5)  [unwired: 8 in]
        n64 = global read "TrajectoryGlobals.vi" "TwoPieceCenterFwd"() -> (w120:T6)
        n65 = call <vilib>:"Conv_Radians_Deg.vi"("Radians"=w105) -> ("Degrees"=w116:dbl)  [unwired: 10 in]
        n66 = call "TrajectoryExecuteRelative.vi"("Init"=w106, "End Relative\nOrientation Deg"=w116, "Trajectory"=w120) -> ("Done"=w111:bool, "Chassis Velocity Target Met,Met,Rad"=w124:T11)  [unwired: 6 in, 1 out]
        n67 = Or(x=w110, y=w111) -> (x .or. y?=w109:bool)
        n68 = call <vilib>:"ChassisSpeeds_GetXYOmega.vi"("CHASSIS"=w124) -> ("vAngular"=w127:dbl, "vY"=w126:dbl, "vX"=w125:dbl)  [unwired: 8 in]
        n69 = case shown="True" w111 {
          tunnel: w125 -> [w130 _]
          tunnel: w126 -> [w129 _]
          tunnel: w127 -> [w128 _]
          tunnel: [w130 w132] -> w123
          tunnel: [w129 w132] -> w122
          tunnel: [w128 w132] -> w121
          tunnel: [_ TRUE ("First Time")] -> w107
          frame False {
          }
          frame True {
            w132 = 0.0 ("XSpeedDemand")
          }
        }
        n70 = call "Check Step Complete.vi"("Move Complete"=w109, "Main Array in"=w113) -> ("Main Array iout"=w112:T5)  [unwired: 9 in]
        n71 = call <vilib>:"Conv_Meters_Feet.vi"("Meters"=w123) -> ("Feet"=w119:dbl)  [unwired: 10 in]
        n72 = call <vilib>:"Conv_Meters_Feet.vi"("Meters"=w122) -> ("Feet"=w118:dbl)  [unwired: 10 in]
        n73 = call <vilib>:"Conv_Radians_Deg.vi"("Radians"=w121) -> ("Degrees"=w117:dbl)  [unwired: 10 in]
        n74 = Bundle By Name(cluster=w112, "First Time"=w107) -> (w108:T5)
      }
      frame "Drive Turn" {
        w136 = 0.0 ("Result")
        n75 = Unbundle By Name(w141) -> ("Current Step.Dist"=w139:dbl, "Current Step.MaxSpeed (ft/s)"=w138:dbl, "First Time"=w140:bool)
        n76 = call "Check if Timed Out).vi"("Main Array in"=w141) -> ("Timed Out"=w135:bool, "Main Array out"=w143:T5)  [unwired: 9 in]
        n77 = call "ActTurn.vi"("FirstTime"=w140, "MaxSpeed (ft/s)"=w138, "Degrees"=w139) -> ("RotationSpeedDemand Deg/Sec"=w137:dbl, "Done"=w134:bool)  [unwired: 7 in]
        n78 = Or(x=w135, y=w134) -> (x .or. y?=w133:bool)
        n79 = call "Check Step Complete.vi"("Move Complete"=w133, "Main Array in"=w143) -> ("Main Array iout"=w142:T5)  [unwired: 9 in]
      }
      frame "Move Arm" {
        w145 = 0.0 ("Result")
        n80 = Unbundle By Name(w144) -> ("TimeOut (s)"=w150:dbl, "Current Step.ArmSetpoints"=w146:T1)
        n81 = call "Check if Timed Out).vi"("Time out"=w150, "Main Array in"=w144) -> ("Timed Out"=w149:bool, "Main Array out"=w152:T5)  [unwired: 8 in]
        n82 = call "ShoulderAtSetpoint.vi"("SholdrSetpoints"=w146) -> ("AtSetpoint"=w147:bool)  [unwired: 10 in]
        n83 = Or(x=w149, y=w147) -> (x .or. y?=w148:bool)
        n84 = call "Check Step Complete.vi"("Move Complete"=w148, "Main Array in"=w152) -> ("Main Array iout"=w151:T5)  [unwired: 9 in]
      }
      frame "Send Bool CMD" {
        w154 = 0.0 ("Result")
        n85 = Unbundle By Name(w153) -> ("TimeOut (s)"=w158:dbl, "Current Step.CMD"=w159:string)
        n86 = call "Check if Timed Out).vi"("Time out"=w158, "Main Array in"=w153) -> ("Timed Out"=w155:bool, "Main Array out"=w157:T5)  [unwired: 8 in]
        n87 = call <vilib>:"BoolCmd_Send.vi"("Command Name"=w159) -> ()  [unwired: 10 in, 1 out]
        n88 = call "Check Step Complete.vi"("Move Complete"=w155, "Main Array in"=w157) -> ("Main Array iout"=w156:T5)  [unwired: 9 in]
      }
      frame "Set Target" {
      }
      frame "Shoot" {
        n89 = Unbundle By Name(w161) -> ("TimeOut (s)"=w165:dbl)
        n90 = call "EminemGetCommandReady.vi"() -> ("BoxCommandReady"=w162:bool)  [unwired: 11 in]
        n91 = call "Check if Timed Out).vi"("Time out"=w165, "Main Array in"=w161) -> ("Timed Out"=w164:bool, "Main Array out"=w167:T5)  [unwired: 8 in]
        n92 = Or(x=w164, y=w162) -> (x .or. y?=w163:bool)
        n93 = call "Check Step Complete.vi"("Move Complete"=w163, "Main Array in"=w167) -> ("Main Array iout"=w166:T5)  [unwired: 9 in]
      }
      frame "Intake" {
      }
      frame "Exit" {
        w169 = 0.0 ("Result")
      }
    }
    n94 = call "DriveSetSpeedDemand.vi"("ASpeedDemand (d/s)"=w63, "YSpeedDemand (ft/s)"=w64, "XSpeedDemand (ft/s)"=w65) -> ()  [unwired: 9 in]
  }
